vi "Serialize Core.vi"(8 "error in (no error)":errorcluster, 11 "Serializable Message in":refnum<class "echo reply Msg.lvclass">) -> (0 "error out":errorcluster, 2 "Serialized Message":string)   [LabVIEW 2020, in "Chat Window.lvlib" / "echo reply Msg.lvclass"]
uses:
  echo reply Msg.lvclass
  echo reply Msg.lvclass/echo reply Msg.ctl
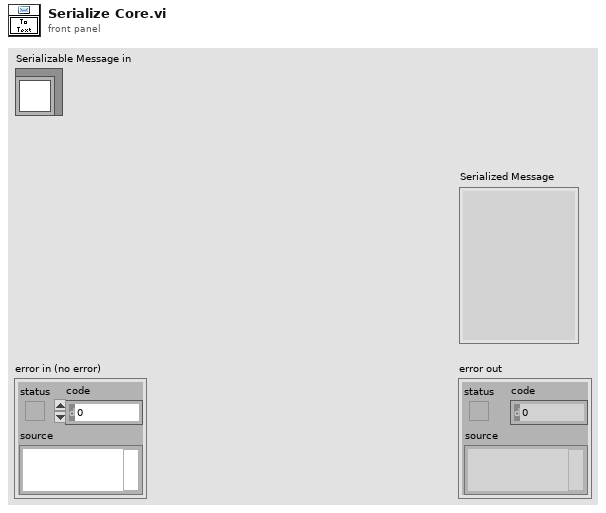
[diagram p1: front panel]
types:
  T1 = cluster{"Message":string, "id":string, "exec_time":i32}
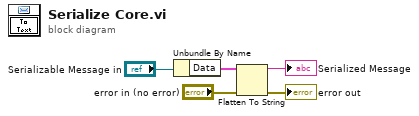
[diagram p0: block diagram]
diagram:
  n1 = Unbundle By Name("Serializable Message in") -> ("Data"=w2:T1)
  n2 = Flatten To String(anything=w2, error in (no error)="error in (no error)") -> (data string=→"Serialized Message":string, error out=→"error out":errorcluster)  [unwired: 2 in, 1 out]
